vi "串口配置.vi"(8 "PORT":string="1001", 9 "IP":string="127.0.0.1", 11 "请选择串口:":refnum<visa-resource-name>) -> (0 "PORT 2":string="1001", 1 "IP 2":string="127.0.0.1", 2 "确认 2":bool, 3 "VISA资源名称 2":refnum<visa-resource-name>, 4 "MB通信方式选择 2":enum16{"串口", "TCP"}(ring))   [LabVIEW 2016, in "斯坦道氨氮.lvlib"]
panel:
  in  "MB通信方式选择":enum16{"串口", "TCP"}(ring)
  in  "取消":bool
  in  "确认":bool
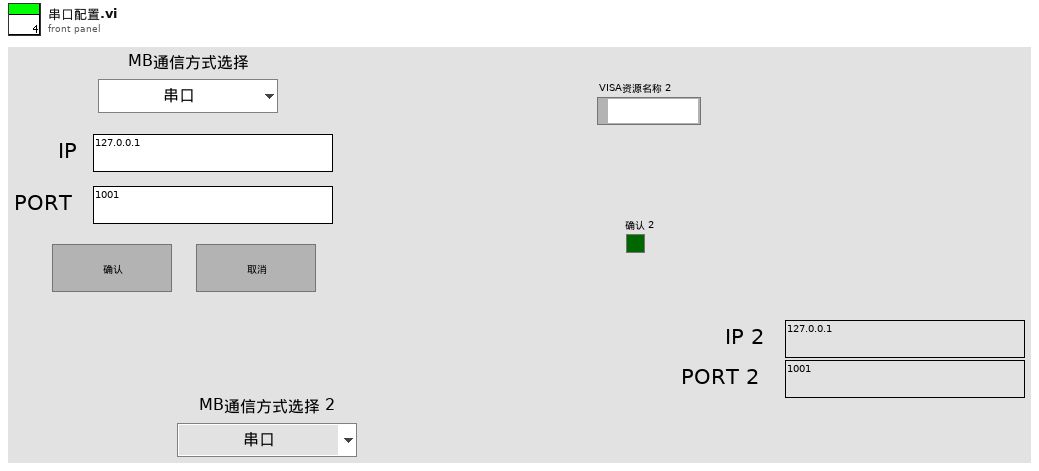
[diagram p1: front panel]
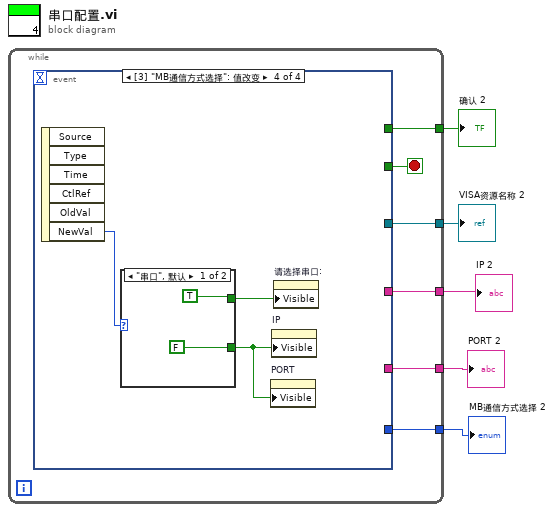
[diagram p0: block diagram]
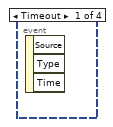
[diagram p2: hidden frame]
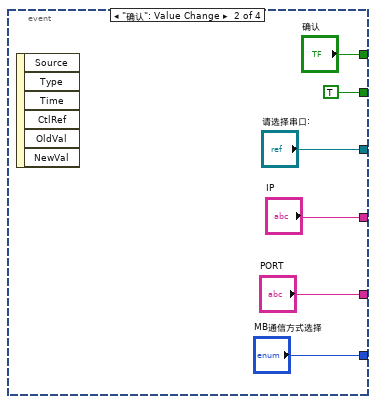
[diagram p3: hidden frame]
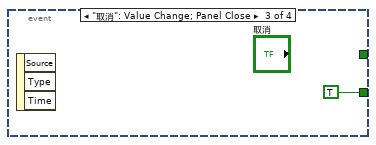
[diagram p4: hidden frame]
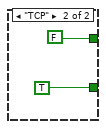
[diagram p5: hidden frame]
diagram:
  n1 = while {
    tunnel: [w11] -> w5
    tunnel: [w9] -> w4
    tunnel: [w8] -> w3
    tunnel: [w7] -> w2
    tunnel: [w6] -> w1
    stop <- w10 stop-if-true
    n2 = event shown="[3] \"MB通信方式选择\": 值改变" {
      selector: _ -> [_ _ _ _]
      dyn-events: _ -> [_ _ _ _]
      timeout: _ -> [_ _ _ _]
      tunnel: [_ "请选择串口:" _ _] -> w11
      tunnel: [_ TRUE TRUE _] -> w10
      tunnel: [_ "确认" _ _] -> w9
      tunnel: [_ "IP" _ _] -> w8
      tunnel: [_ "PORT" _ _] -> w7
      tunnel: [_ "MB通信方式选择" _ _] -> w6
      event Timeout {
        n3 = event-data() -> ()  [unwired: 1 in, 3 out]
      }
      event "确认": Value Change {
        n4 = event-data() -> ()  [unwired: 1 in, 6 out]
      }
      event "取消": Value Change; Panel Close {
        n5 = event-data() -> ()  [unwired: 1 in, 3 out]
      }
      event "MB通信方式选择": Value Change {
        n6 = event-data() -> ("NewVal"=w19:enum16{"串口", "TCP"})  [unwired: 1 in, 5 out]
        n7 = case shown="\"串口\", 默认" w19 {
          tunnel: [FALSE ("可见") TRUE ("可见")] -> w20
          tunnel: [TRUE ("可见") FALSE ("可见")] -> w21
          frame "串口", Default {
          }
          frame "TCP" {
          }
        }
        n8 = property on="PORT" class="Str"("Visible"=w20) -> ()  [unwired: 2 in, 2 out]
        n9 = property on="IP" class="Str"("Visible"=w20) -> ()  [unwired: 2 in, 2 out]
        n10 = property on="请选择串口:" class="VISAName"("Visible"=w21) -> ()  [unwired: 2 in, 2 out]
      }
    }
  }
  "VISA资源名称 2" <- w5
  "确认 2" <- w4
  "IP 2" <- w3
  "PORT 2" <- w2
  "MB通信方式选择 2" <- w1
